vi "subvi_RemNotAlphaNum.vi"(0 "In_String":string) -> (1 "clan_String":string, 2 "Basura":bool)   [LabVIEW 2019]
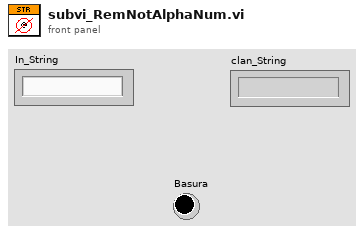
[diagram p1: front panel]
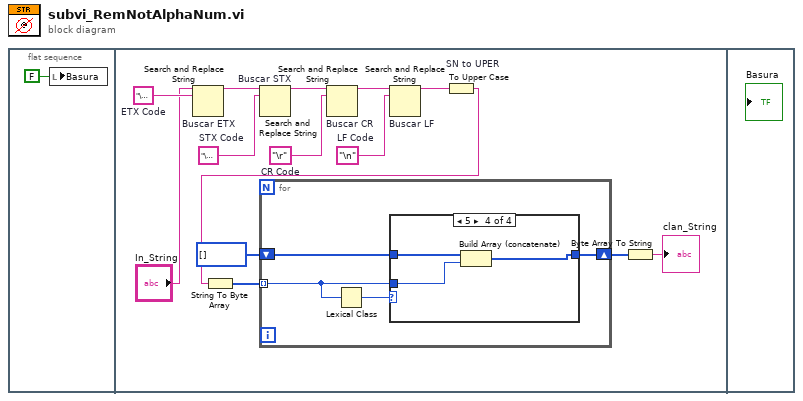
[diagram p0: block diagram]
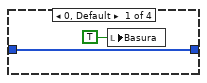
[diagram p2: hidden frame]
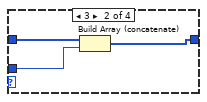
[diagram p3: hidden frame]
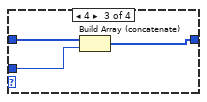
[diagram p4: hidden frame]
diagram:
  n1 = flat-sequence {
    frame #0 {
      n2 = local write "Basura"(FALSE ("Basura")) -> ()
    }
    frame #1 {
      w7 = "\n"  # LF Code
      w8 = "\r"  # CR Code
      w10 = "\u0003"  # ETX Code
      w9 = "\u0002"  # STX Code
      n3 = Search and Replace String "Buscar ETX"(input string="In_String", search string=w10) -> (result string=w11:string)  [unwired: 6 in, 3 out]
      n4 = Search and Replace String "Buscar STX"(input string=w11, search string=w9) -> (result string=w5:string)  [unwired: 6 in, 3 out]
      n5 = Search and Replace String "Buscar CR"(input string=w5, search string=w8) -> (result string=w6:string)  [unwired: 6 in, 3 out]
      n6 = Search and Replace String "Buscar LF"(input string=w6, search string=w7) -> (result string=w4:string)  [unwired: 6 in, 3 out]
      n7 = To Upper Case "SN to UPER"(1:w4) -> (0:w2:string)
      n8 = String To Byte Array(string=w2) -> (unsigned byte array=w13:u8[])
      n9 = for {
        tunnel: w13 -> [w19] mode=indexing
        shift-right: [w17] -> w15
        shift-left: i32[] [] -> [w18]
        n10 = Lexical Class(1:w19) -> (0:w16:i16)
        n11 = case shown="5" w16 {
          tunnel: w18 -> [w21 w24 w27 w28]
          tunnel: w19 -> [_ w23 w26 w29]
          tunnel: [w21 w22 w25 w30] -> w17
          frame 0, Default {
            n12 = local write "Basura"(TRUE ("Basura")) -> ()
          }
          frame 3 {
            n13 = Build Array (concatenate)(w24, w23) -> (w22:i32[])
          }
          frame 4 {
            n14 = Build Array (concatenate)(w27, w26) -> (w25:i32[])
          }
          frame 5 {
            n15 = Build Array (concatenate)(w28, w29) -> (w30:i32[])
          }
        }
      }
      n16 = Byte Array To String(unsigned byte array=w15) -> (string=→"clan_String":string)
    }
    frame #2 {
    }
  }
